vi "XNET.Settings.vi"(6 "Action":enum8{"Get", "Set"}(ring), 8 "error in (no error)":errorcluster, 10 "XNET Settings":T1={"Database"="", "Cluster"="", "Port"="", "Baud rate [Bd]"=500000, "Termination"=1, "CAN I/O Mode"=0, "FD Baud rate [Bd]"=500000, "Priority"=100, "Use Legacy"=FALSE} {"CAN I/O Mode" items=["CAN 2.0", "CAN FD", "CAN FD+BRS"]; "Termination" items=["Off", "On"]}, 11 "Parent Ref in":T2 format="%.0x") -> (0 "error out":errorcluster, 2 "XNET Settings":T1={"Database"="", "Cluster"="", "Port"="", "Baud rate [Bd]"=500000, "Termination"=1, "CAN I/O Mode"=0, "FD Baud rate [Bd]"=500000, "Priority"=100, "Use Legacy"=FALSE} {"CAN I/O Mode" items=["CAN 2.0", "CAN FD", "CAN FD+BRS"]; "Termination" items=["Off", "On"]}, 3 "Item Ref out":T2 format="%.0x")   [LabVIEW 2015, in "Protection and Rolling Counter Addon System Explorer.lvlib"]
uses:
  Protection and Rolling Counter Addon System Explorer.lvlib
  Shared/Types/XNET Settings.ctl
  <vilib>/NI Veristand/Custom Device API/Custom Device Item Ref.ctl
  Shared/SubVIs/GUID Lookup.vi
  <vilib>/NI/NI VeriStand Advanced SysDef API/_SubVIs/SysDef.Property.Set.String.vi
  <vilib>/NI/NI VeriStand Advanced SysDef API/_SubVIs/SysDef.Property.Set.Variant.vi
  <vilib>/NI/NI VeriStand Advanced SysDef API/_SubVIs/SysDef.Property.Set.U32.vi
  <vilib>/NI/NI VeriStand Advanced SysDef API/_SubVIs/SysDef.Property.Set.I32.vi
  <vilib>/NI/NI VeriStand Advanced SysDef API/_SubVIs/SysDef.Property.Set.Boolean.vi
  <vilib>/NI Veristand/Custom Device API/Get Item Property (String).vi
  <vilib>/NI Veristand/Custom Device API/Get Item Property (Variant).vi
  <vilib>/NI Veristand/Custom Device API/Get Item Property (U32).vi
  <vilib>/NI Veristand/Custom Device API/Get Item Property (I32).vi
  <vilib>/NI Veristand/Custom Device API/Get Item Property (Boolean).vi
  <vilib>/NI VeriStand/Custom Device API/Custom Device API.lvlib
  <vilib>/NI/NI VeriStand Advanced SysDef API/SysDef API/Advanced System Definition.lvlib
  Shared/Protection and Rolling Counter Addon Shared.lvlib
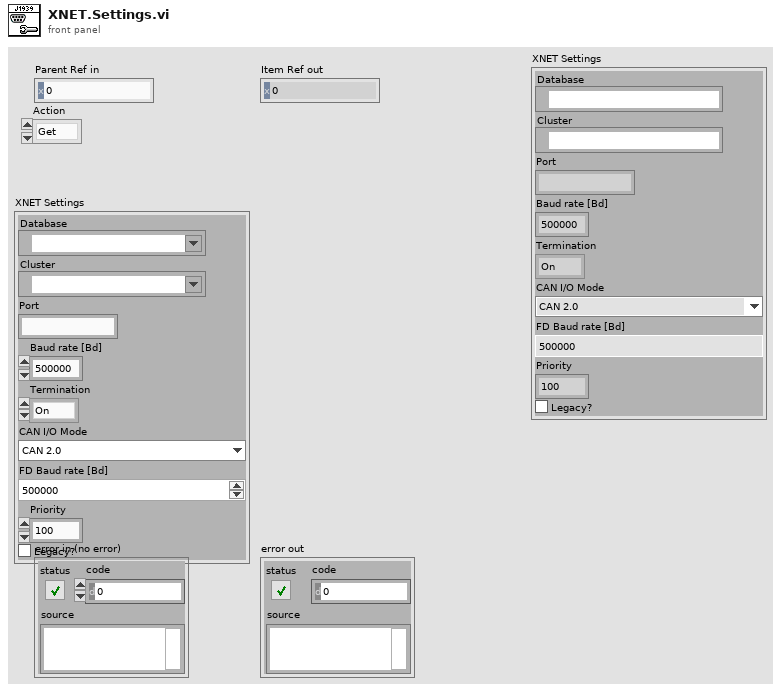
[diagram p1: front panel]
types:
  T1 = typedef "Protection and Rolling Counter Addon Shared.lvlib/XNET Settings.ctl" = cluster{"Database":refnum<k21>, "Cluster":refnum<k21>, "Port":string, "Baud rate [Bd]":u64, "Termination":u32, "CAN I/O Mode":u32, "FD Baud rate [Bd]":u64, "Priority":i32, "Use Legacy":bool}
  T2 = typedef "Custom Device API.lvlib/Custom Device Item Ref.ctl" = u64
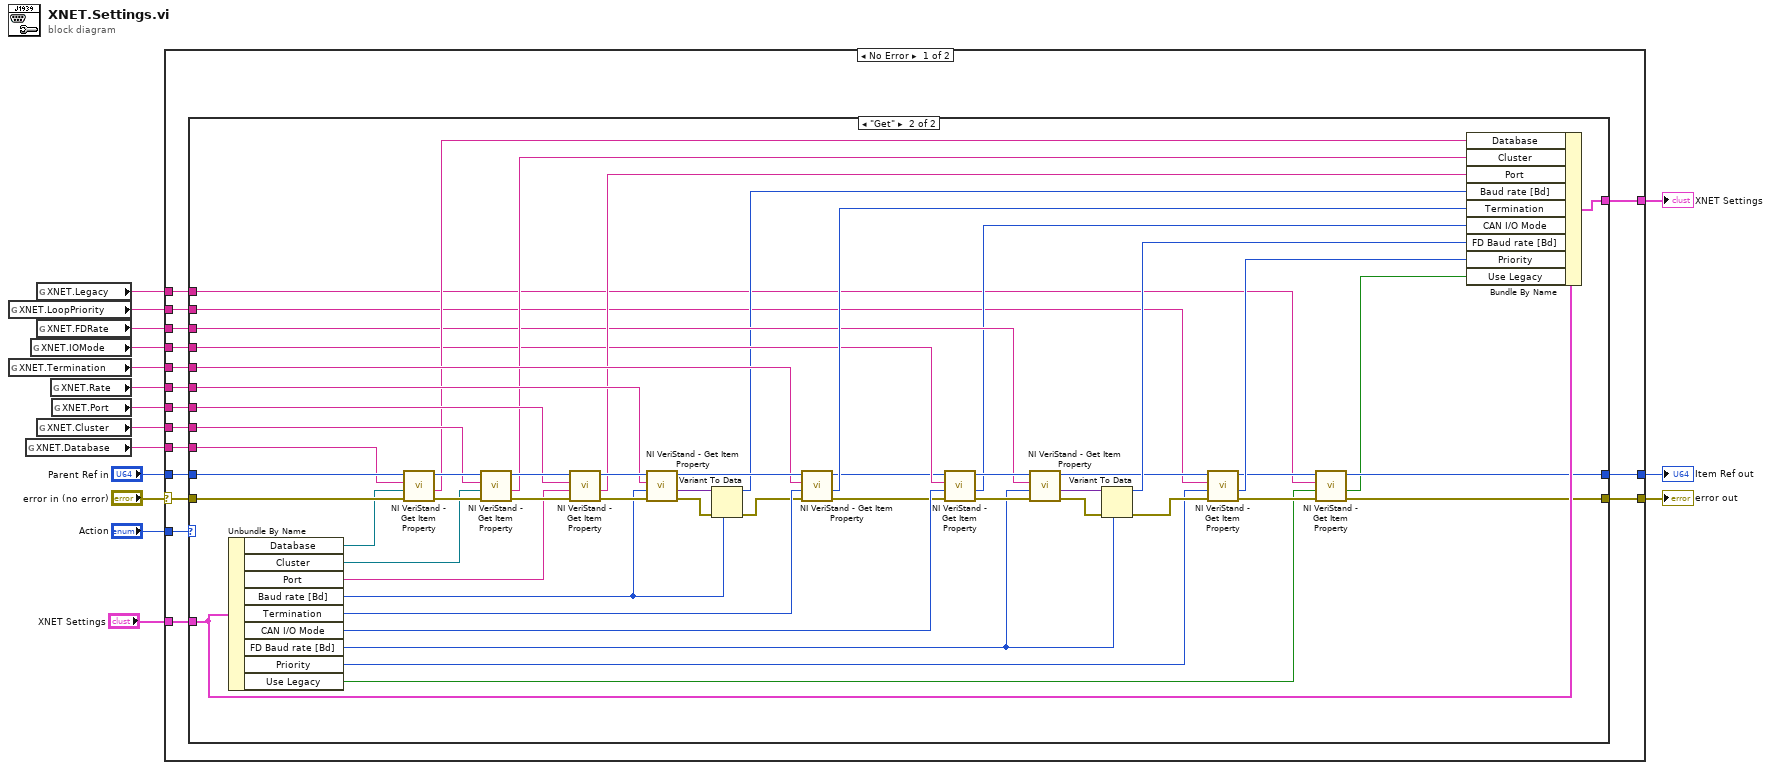
[diagram p0: block diagram]
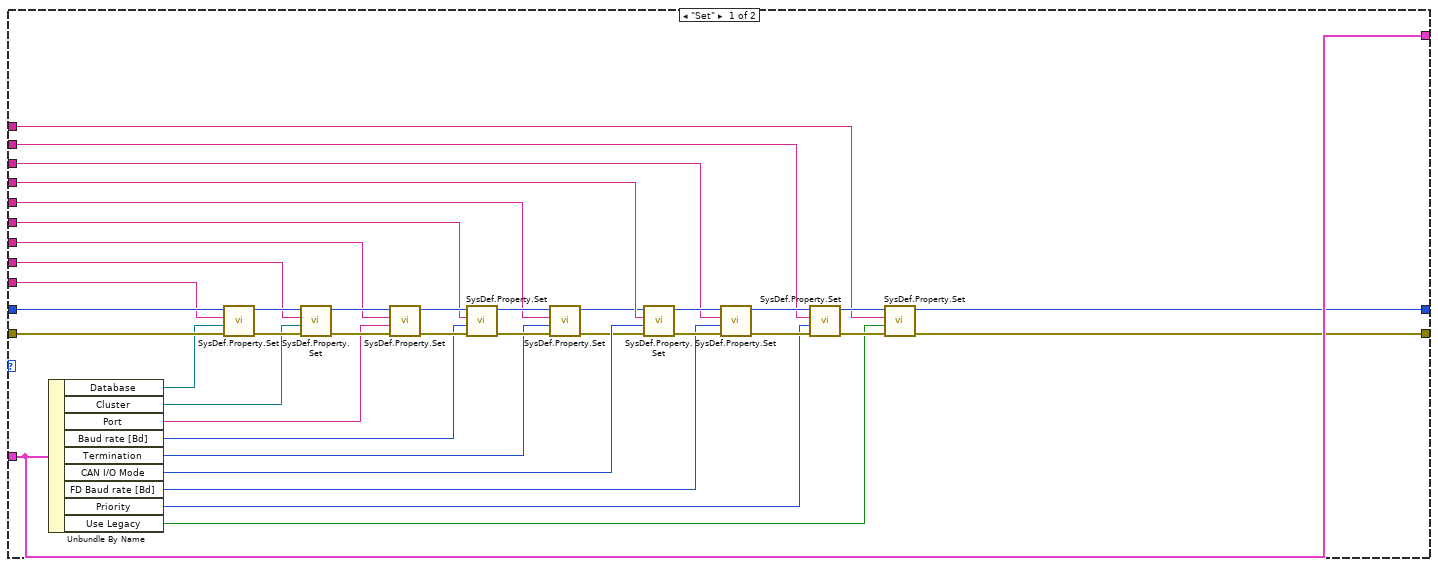
[diagram p2: hidden frame]
diagram:
  n1 = global read "GUID Lookup.vi" "XNET.LoopPriority"() -> (w2:string)
  n2 = global read "GUID Lookup.vi" "XNET.Termination"() -> (w5:string)
  n3 = global read "GUID Lookup.vi" "XNET.Database"() -> (w9:string)
  n4 = global read "GUID Lookup.vi" "XNET.IOMode"() -> (w4:string)
  n5 = global read "GUID Lookup.vi" "XNET.Legacy"() -> (w1:string)
  n6 = global read "GUID Lookup.vi" "XNET.FDRate"() -> (w3:string)
  n7 = global read "GUID Lookup.vi" "XNET.Cluster"() -> (w8:string)
  n8 = global read "GUID Lookup.vi" "XNET.Rate"() -> (w6:string)
  n9 = global read "GUID Lookup.vi" "XNET.Port"() -> (w7:string)
  n10 = case shown="No Error" "error in (no error)" {
    selector: "error in (no error)" -> [w23 w127]
    tunnel: "Parent Ref in" -> [w32 w126]
    tunnel: w9 -> [w31 _]
    tunnel: "XNET Settings" -> [w30 w125]
    tunnel: [w29 w127] -> w14
    tunnel: [w28 w126] -> w13
    tunnel: w8 -> [w27 _]
    tunnel: w7 -> [w26 _]
    tunnel: w5 -> [w25 _]
    tunnel: w6 -> [w24 _]
    tunnel: "Action" -> [w22 _]
    tunnel: [w21 w125] -> w10
    tunnel: w4 -> [w20 _]
    tunnel: w3 -> [w19 _]
    tunnel: w2 -> [w18 _]
    tunnel: w1 -> [w17 _]
    frame No Error {
      n11 = case shown="\"Get\"" w22 {
        tunnel: w32 -> [w71 w124]
        tunnel: w31 -> [w70 w123]
        tunnel: w30 -> [w52 w106]
        tunnel: [w35 w75] -> w29
        tunnel: [w36 w76] -> w28
        tunnel: w27 -> [w57 w115]
        tunnel: w26 -> [w56 w114]
        tunnel: w25 -> [w55 w113]
        tunnel: w24 -> [w54 w112]
        tunnel: w23 -> [w53 w111]
        tunnel: [w52 w101] -> w21
        tunnel: w20 -> [w48 w97]
        tunnel: w19 -> [w47 w96]
        tunnel: w18 -> [w39 w81]
        tunnel: w17 -> [w34 w73]
        frame "Set" {
          n12 = Unbundle By Name(w52) -> ("Database"=w51:refnum<k21>, "Cluster"=w61:refnum<k21>, "Port"=w60:string, "Baud rate [Bd]"=w59:u64, "Termination"=w58:u32, "CAN I/O Mode"=w46:u32, "FD Baud rate [Bd]"=w45:u64, "Priority"=w40:i32, "Use Legacy"=w33:bool)
          n13 = call-poly <vilib>:"SysDef.Property.Set.vi"("error in (no error)"=w53, "Value"=w51, "Property Name"=w70, "nodeID"=w71) -> ("error out"=w67:errorcluster, "nodeID out"=w66:u64)  [unwired: 6 in]
          n14 = call-poly <vilib>:"SysDef.Property.Set.vi"("error in (no error)"=w67, "Value"=w61, "Property Name"=w57, "nodeID"=w66) -> ("error out"=w68:errorcluster, "nodeID out"=w69:u64)  [unwired: 6 in]
          n15 = call-poly <vilib>:"SysDef.Property.Set.vi"("error in (no error)"=w68, "Value"=w60, "Property Name"=w56, "nodeID"=w69) -> ("error out"=w63:errorcluster, "nodeID out"=w62:u64)  [unwired: 6 in]
          n16 = call-poly <vilib>:"SysDef.Property.Set.vi"("error in (no error)"=w63, "Value"=w59, "Property Name"=w54, "nodeID"=w62) -> ("error out"=w64:errorcluster, "nodeID out"=w65:u64)  [unwired: 6 in]
          n17 = call-poly <vilib>:"SysDef.Property.Set.vi"("error in (no error)"=w64, "Value"=w58, "Property Name"=w55, "nodeID"=w65) -> ("error out"=w44:errorcluster, "nodeID out"=w43:u64)  [unwired: 6 in]
          n18 = call-poly <vilib>:"SysDef.Property.Set.vi"("error in (no error)"=w44, "Value"=w46, "Property Name"=w48, "nodeID"=w43) -> ("error out"=w50:errorcluster, "nodeID out"=w49:u64)  [unwired: 6 in]
          n19 = call-poly <vilib>:"SysDef.Property.Set.vi"("error in (no error)"=w50, "Value"=w45, "Property Name"=w47, "nodeID"=w49) -> ("error out"=w42:errorcluster, "nodeID out"=w41:u64)  [unwired: 6 in]
          n20 = call-poly <vilib>:"SysDef.Property.Set.vi"("error in (no error)"=w42, "Value"=w40, "Property Name"=w39, "nodeID"=w41) -> ("error out"=w38:errorcluster, "nodeID out"=w37:u64)  [unwired: 6 in]
          n21 = call-poly <vilib>:"SysDef.Property.Set.vi"("error in (no error)"=w38, "Value"=w33, "Property Name"=w34, "nodeID"=w37) -> ("error out"=w35:errorcluster, "nodeID out"=w36:u64)  [unwired: 6 in]
        }
        frame "Get" {
          n22 = Unbundle By Name(w106) -> ("Database"=w110:refnum<k21>, "Cluster"=w109:refnum<k21>, "Port"=w108:string, "Baud rate [Bd]"=w87:u64, "Termination"=w107:u32, "CAN I/O Mode"=w98:u32, "FD Baud rate [Bd]"=w93:u64, "Priority"=w80:i32, "Use Legacy"=w72:bool)
          n23 = call-poly <vilib>:"NI VeriStand - Get Item Property.vi"("error in (no error)"=w111, "Default Value"=w110, "Property Name"=w123, "Item Ref in"=w124) -> ("error out"=w120:errorcluster, "Value"=w105:string, "Item Ref out"=w119:T2)  [unwired: 4 in, 1 out]
          n24 = call-poly <vilib>:"NI VeriStand - Get Item Property.vi"("error in (no error)"=w120, "Default Value"=w109, "Property Name"=w115, "Item Ref in"=w119) -> ("error out"=w121:errorcluster, "Value"=w104:string, "Item Ref out"=w122:T2)  [unwired: 4 in, 1 out]
          n25 = call-poly <vilib>:"NI VeriStand - Get Item Property.vi"("error in (no error)"=w121, "Default Value"=w108, "Property Name"=w114, "Item Ref in"=w122) -> ("error out"=w117:errorcluster, "Value"=w103:string, "Item Ref out"=w116:T2)  [unwired: 4 in, 1 out]
          n26 = call-poly <vilib>:"NI VeriStand - Get Item Property.vi"("error in (no error)"=w117, "Default Value"=w87, "Property Name"=w112, "Item Ref in"=w116) -> ("error out"=w84:errorcluster, "Value"=w86:variant, "Item Ref out"=w118:T2)  [unwired: 4 in, 1 out]
          n27 = Variant To Data(error in=w84, type=w87, Variant=w86) -> (data=w85:u64, error out=w88:errorcluster)
          n28 = call-poly <vilib>:"NI VeriStand - Get Item Property.vi"("error in (no error)"=w88, "Default Value"=w107, "Property Name"=w113, "Item Ref in"=w118) -> ("error out"=w89:errorcluster, "Value"=w102:u32, "Item Ref out"=w90:T2)  [unwired: 4 in, 1 out]
          n29 = call-poly <vilib>:"NI VeriStand - Get Item Property.vi"("error in (no error)"=w89, "Default Value"=w98, "Property Name"=w97, "Item Ref in"=w90) -> ("error out"=w100:errorcluster, "Value"=w95:u32, "Item Ref out"=w99:T2)  [unwired: 4 in, 1 out]
          n30 = call-poly <vilib>:"NI VeriStand - Get Item Property.vi"("error in (no error)"=w100, "Default Value"=w93, "Property Name"=w96, "Item Ref in"=w99) -> ("error out"=w92:errorcluster, "Value"=w94:variant, "Item Ref out"=w82:T2)  [unwired: 4 in, 1 out]
          n31 = Variant To Data(error in=w92, type=w93, Variant=w94) -> (data=w91:u64, error out=w83:errorcluster)
          n32 = call-poly <vilib>:"NI VeriStand - Get Item Property.vi"("error in (no error)"=w83, "Default Value"=w80, "Property Name"=w81, "Item Ref in"=w82) -> ("error out"=w78:errorcluster, "Value"=w79:i32, "Item Ref out"=w77:T2)  [unwired: 4 in, 1 out]
          n33 = call-poly <vilib>:"NI VeriStand - Get Item Property.vi"("error in (no error)"=w78, "Default Value"=w72, "Property Name"=w73, "Item Ref in"=w77) -> ("error out"=w75:errorcluster, "Value"=w74:bool, "Item Ref out"=w76:T2)  [unwired: 4 in, 1 out]
          n34 = Bundle By Name(cluster=w106, "Database"=w105, "Cluster"=w104, "Port"=w103, "Baud rate [Bd]"=w85, "Termination"=w102, "CAN I/O Mode"=w95, "FD Baud rate [Bd]"=w91, "Priority"=w79, "Use Legacy"=w74) -> (w101:T1)
        }
      }
    }
    frame Error {
    }
  }
  "Item Ref out" <- w13
  "error out" <- w14
  "XNET Settings" <- w10
